vi "DAQmxTasksVI.vi"(8 "error in (no error)":errorcluster, 10 "ControlQueue":refnum<queue>, 11 "DAQmxTaskContainer.lvclass":refnum<class "DAQmxTaskContainer.lvclass">) -> ()   [LabVIEW 2015, in "DAQmxTaskContainer.lvclass"]
uses:
  DAQmxTaskContainer.lvclass
  dependecies/ControlsVIs/Clusters-def/Message types.ctl
  DAQmxTaskContainer.lvclass/DAQmxTaskContainer.ctl
  GeneralFunctionality/GeneralFunctionality.lvclass/GeneralFunctionality.ctl
  Message/Message.lvclass/Message.ctl
  dependecies/ControlsVIs/Clusters-def/Standard Command.ctl
  DAQmxTask.lvclass
  Message/Message.lvclass
  GeneralFunctionality/GeneralFunctionality.lvclass
panel:
  in  "ReInit":bool
  out "Alarm":bool
  in  "divider":i8(knob)=10 min=1 max=20 step=1 scale=1.0..20.0
  out "ELYSE clock pulses":dbl
  out "Received command":string
  in  "DAQmx Tasks":T1(array[cluster])
  out "error out":errorcluster
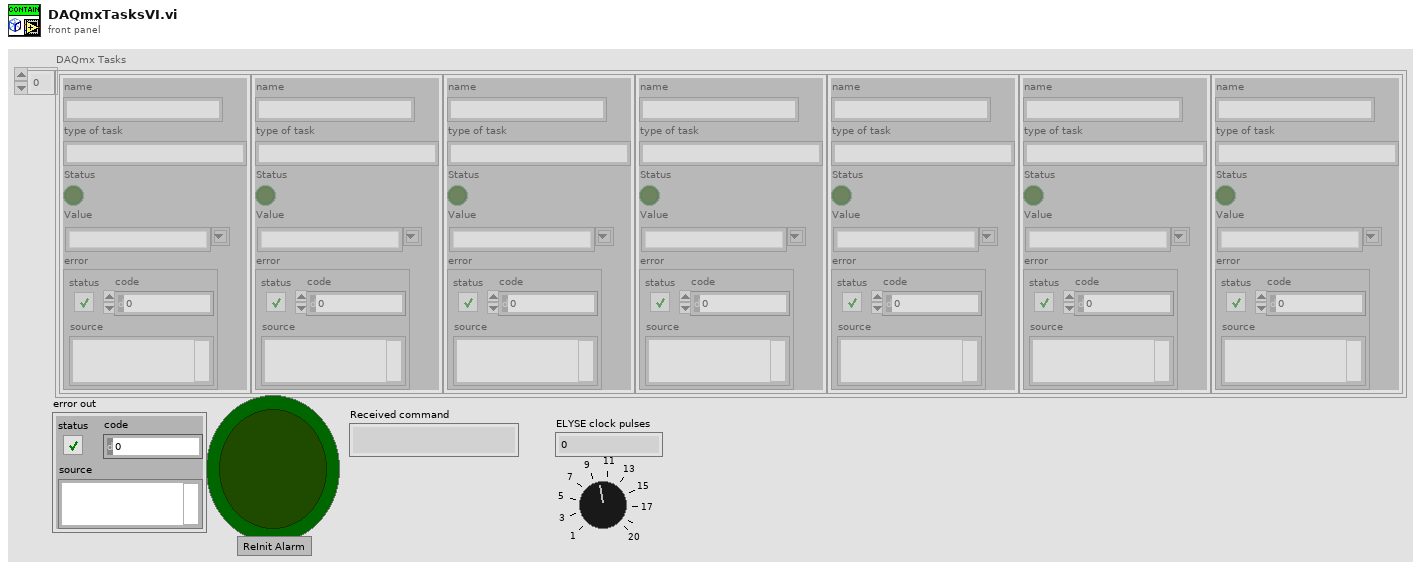
[diagram p1: front panel]
types:
  T1 = cluster{"name":string, "type of task":string, "Status":bool, "Value":string, "error":errorcluster}[]
  T2 = typedef "Message types.ctl" = string
  T3 = typedef "Standard Command.ctl" = cluster{"command":string, "data":variant}
  T4 = cluster{"name":string, "type of task":string, "Status":bool, "Value":string, "error":errorcluster}
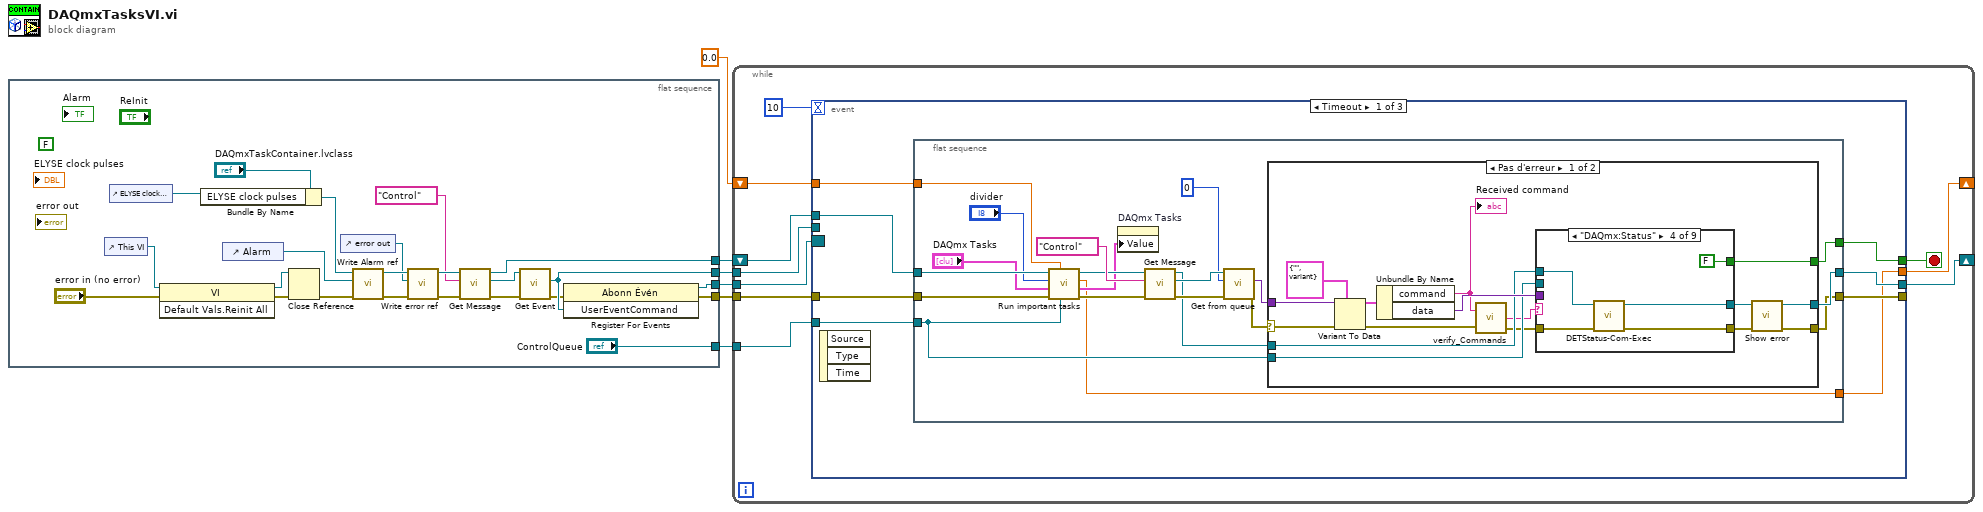
[diagram p0: block diagram]
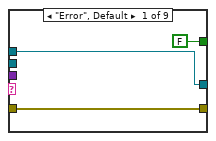
[diagram p2: hidden frame]
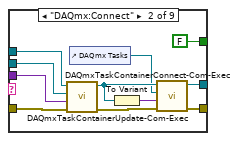
[diagram p3: hidden frame]
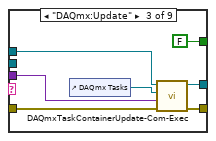
[diagram p4: hidden frame]
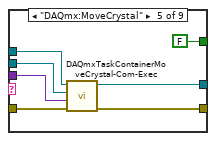
[diagram p5: hidden frame]
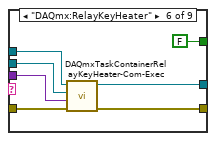
[diagram p6: hidden frame]
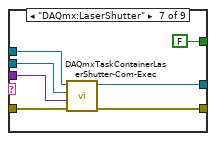
[diagram p7: hidden frame]
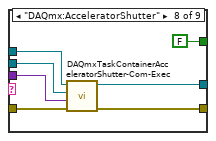
[diagram p8: hidden frame]
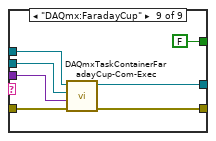
[diagram p9: hidden frame]
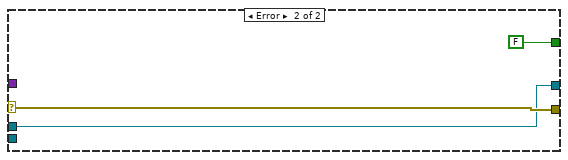
[diagram p10: hidden frame]
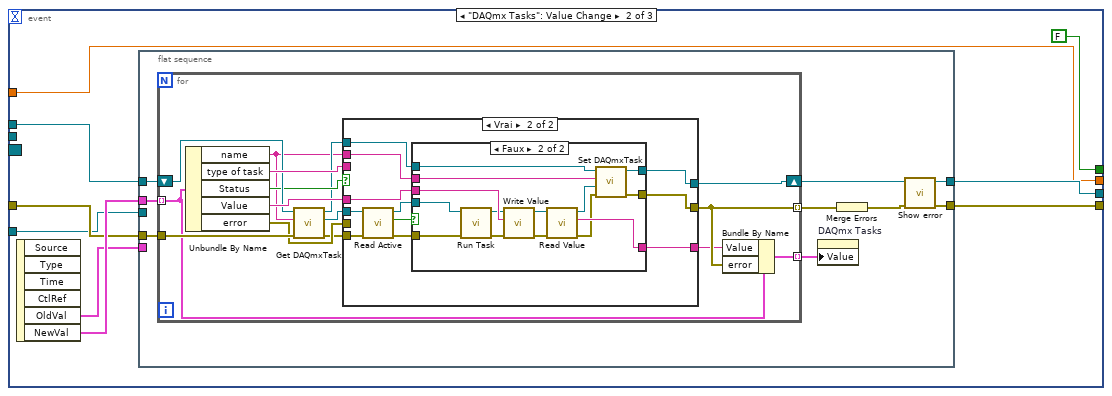
[diagram p11: hidden frame]
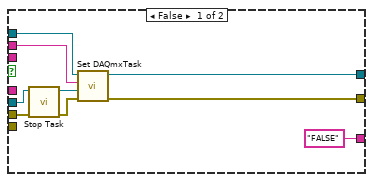
[diagram p12: hidden frame]
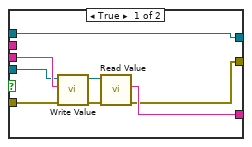
[diagram p13: hidden frame]
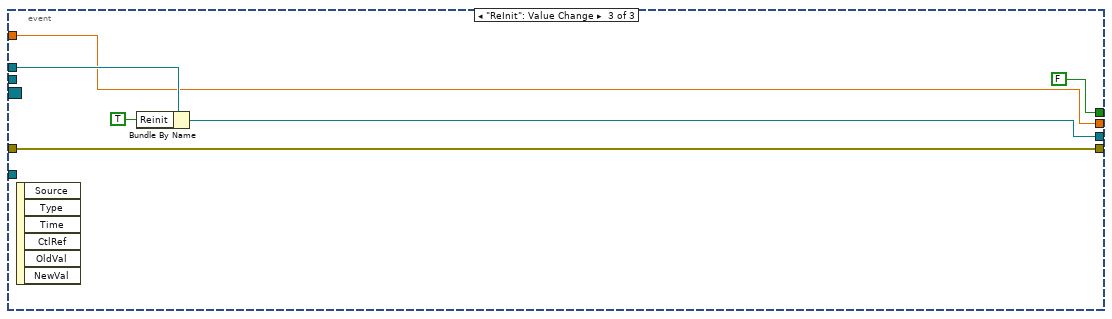
[diagram p14: hidden frame]
diagram:
  n1 = flat-sequence {
    tunnel: [w29] -> w6
    tunnel: [w28] -> w5
    tunnel: ["ControlQueue"] -> w4
    tunnel: [w15] -> w3
    tunnel: [w14] -> w2
    frame #0 {
      (unwired) FALSE ("Clignotant")
      n2 = control-ref of="This VI"() -> (w26:refnum<vi>)
      n3 = control-ref of="ELYSE clock pulses"() -> (w8:refnum<vi>)
      n4 = invoke class="VI" method="Default Vals.Reinit All"(reference=w26, error in="error in (no error)") -> (reference out=w25:refnum<vi>, error out=w27:errorcluster)  [unwired: 1 in, 1 out]
      n5 = Bundle By Name(cluster="DAQmxTaskContainer.lvclass", "ELYSE clock pulses"=w8) -> (w9:refnum<class "DAQmxTaskContainer.lvclass">)
      n6 = control-ref of="Alarm"() -> (w7:refnum<vi>)
      n7 = Close Reference(reference=w25, error in (no error)=w27) -> (error out=w12:errorcluster)
      n8 = control-ref of="error out"() -> (w21:refnum<vi>)
      n9 = call "Write Alarm ref.vi"("error in (no error)"=w12, "Alarm"=w7, "DAQmxTaskContainer in"=w9) -> ("error out"=w23:errorcluster, "DAQmxTaskContainer out"=w22:refnum<class "DAQmxTaskContainer.lvclass">)  [unwired: 7 in]
      n10 = call "Write error ref.vi"("error in (no error)"=w23, "error"=w21, "GeneralFunctionality in"=w22) -> ("error out"=w18:errorcluster, "GeneralFunctionality out"=w17:refnum<class "DAQmxTaskContainer.lvclass">)  [unwired: 7 in]
      n11 = call "Get Message.vi"("error in (no error)"=w18, "Message type"=T2 "Control", "GeneralFunctionality en entrée"=w17) -> ("error out"=w19:errorcluster, "Message.lvclass"=w20:refnum<class "Message.lvclass">, "GeneralFunctionality en sortie"=w14:refnum<class "DAQmxTaskContainer.lvclass">)  [unwired: 6 in]
      n12 = call "Get Event.vi"("error in (no error)"=w19, "Message en entrée"=w20) -> ("error out"=w11:errorcluster, "UserEventCommand"=w15:refnum<user-event>)  [unwired: 7 in, 1 out]
      n13 = register-events(error in=w11, w15) -> (reference out=w29:refnum<event-registration>, error out=w28:errorcluster)  [unwired: 1 in]
    }
  }
  n14 = while {
    tunnel: w6 -> [w39]
    tunnel: w5 -> [w38]
    shift-right: [w36] -> _
    shift-left: w2 -> [w37]
    tunnel: w4 -> [w35]
    tunnel: w3 -> [w33]
    shift-right: [w30] -> _
    shift-left: 0.0 -> [w31]
    stop <- w32 stop-if-true
    n15 = event shown="[0] Timeout" {
      selector: w39 -> [_ _ _]
      dyn-events: _ -> [_ _ _]
      timeout: 10 -> [_ _ _]
      tunnel: [w42 w153 w228] -> _
      tunnel: w38 -> [w44 w155 w228]
      tunnel: w37 -> [w45 w151 w226]
      tunnel: [w43 w152 w225] -> w36
      tunnel: w35 -> [w46 w154 _]
      tunnel: [w47 FALSE ("NewVal") FALSE ("NewVal")] -> w32
      tunnel: w33 -> [_ _ _]
      tunnel: w31 -> [w41 w148 w223]
      tunnel: [w40 w148 w223] -> w30
      event Timeout {
        n16 = event-data() -> ()  [unwired: 1 in, 3 out]
        n17 = flat-sequence {
          tunnel: [w62] -> w47
          tunnel: [w61] -> w43
          tunnel: [w60] -> w42
          tunnel: w46 -> [w53]
          tunnel: w45 -> [w57]
          tunnel: w44 -> [w55]
          tunnel: w41 -> [w49]
          tunnel: [w48] -> w40
          frame #0 {
            n18 = call "Run important tasks.vi"("ControlQueue"=w53, "pulses previous"=w49, "error in (no error)"=w55, "DAQmx Tasks"="DAQmx Tasks", "divider"="divider", "DAQmxTaskContainer in"=w57) -> ("error out"=w54:errorcluster, "DAQmx Tasks out"=w50:T1, "pulses"=w48:dbl, "DAQmxTaskContainer out"=w56:refnum<class "DAQmxTaskContainer.lvclass">)  [unwired: 2 in]
            n19 = property on="DAQmx Tasks" class="Arr (strict)"("Value"=w50) -> ()  [unwired: 2 in, 2 out]
            n20 = call "Get Message.vi"("error in (no error)"=w54, "Message type"=T2 "Control", "GeneralFunctionality en entrée"=w56) -> ("error out"=w67:errorcluster, "Message.lvclass"=w66:refnum<class "Message.lvclass">, "GeneralFunctionality en sortie"=w58:refnum<class "DAQmxTaskContainer.lvclass">)  [unwired: 6 in]
            n21 = call "Get from queue.vi"("error in (no error)"=w67, "timeout in ms (-1)"=0, "Message in"=w66) -> ("error out"=w64:errorcluster, "Data"=w63:variant)  [unwired: 6 in, 1 out]
            n22 = case shown="Pas d'erreur" w64 {
              selector: w64 -> [w81 w146]
              tunnel: w63 -> [w80 _]
              tunnel: [w75 w146] -> w60
              tunnel: [w79 FALSE] -> w62
              tunnel: [w76 w145] -> w61
              tunnel: w58 -> [w77 w145]
              tunnel: w53 -> [w73 _]
              frame No Error {
                n23 = Variant To Data(error in=w81, type=T3 {"command"="", "data"=variant} ("input cluster"), Variant=w80) -> (data=w83:T3, error out=w71:errorcluster)
                n24 = Unbundle By Name(w83) -> ("command"=w68:string, "data"=w78:variant)
                "Received command" <- w68
                n25 = call "verify_Commands.vi"("Command"=w68, "error in"=w71) -> ("Command out"=w69:string, "error out"=w70:errorcluster)  [unwired: 1 out]
                n26 = case shown="\"DAQmx:Status\"" w69 {
                  tunnel: w70 -> [w84 w95 w103 w108 w115 w121 w127 w132 w139]
                  tunnel: [w84 w91 w102 w107 w114 w122 w126 w135 w142] -> w74
                  tunnel: [FALSE FALSE FALSE FALSE FALSE FALSE FALSE FALSE FALSE] -> w79
                  tunnel: [w86 w90 w100 w106 w113 w123 w125 w136 w143] -> w72
                  tunnel: w78 -> [_ w97 w99 _ w116 w120 w128 w133 w140]
                  tunnel: w77 -> [w86 w93 w98 w105 w110 w117 w124 w131 w138]
                  tunnel: w73 -> [_ w96 _ _ w112 w119 w129 w134 w141]
                  frame "Error", Default {
                  }
                  frame "DAQmx:Connect" {
                    n27 = call "DAQmxTaskContainerConnect-Com-Exec.vi"("error in (no error)"=w95, "data"=w97, "ControlQueue"=w96, "DAQmxTaskContainer in"=w93) -> ("error out"=w92:errorcluster, "DAQmxTaskContainer out"=w89:refnum<class "DAQmxTaskContainer.lvclass">)  [unwired: 6 in]
                    n28 = control-ref of="DAQmx Tasks"() -> (w87:refnum<vi>)
                    n29 = To Variant(anything=w89) -> (Variant=w88:variant)
                    n30 = call "DAQmxTaskContainerUpdate-Com-Exec.vi"("error in (no error)"=w92, "data"=w88, "DAQmx Tasks"=w87, "DAQmxTaskContainer in"=w89) -> ("error out"=w91:errorcluster, "DAQmxTaskContainer out"=w90:refnum<class "DAQmxTaskContainer.lvclass">)  [unwired: 6 in]
                  }
                  frame "DAQmx:Update" {
                    n31 = control-ref of="DAQmx Tasks"() -> (w104:refnum<vi>)
                    n32 = call "DAQmxTaskContainerUpdate-Com-Exec.vi"("error in (no error)"=w103, "data"=w99, "DAQmx Tasks"=w104, "DAQmxTaskContainer in"=w98) -> ("error out"=w102:errorcluster, "DAQmxTaskContainer out"=w100:refnum<class "DAQmxTaskContainer.lvclass">)  [unwired: 6 in]
                  }
                  frame "DAQmx:Status" {
                    n33 = call "DETStatus-Com-Exec.vi"("error in (no error)"=w108, "DAQmxTaskContainer in"=w105) -> ("error out"=w107:errorcluster, "DAQmxTaskContainer out"=w106:refnum<class "DAQmxTaskContainer.lvclass">)  [unwired: 8 in]
                  }
                  frame "DAQmx:MoveCrystal" {
                    n34 = call "DAQmxTaskContainerMoveCrystal-Com-Exec.vi"("error in (no error)"=w115, "data"=w116, "ControlQueue"=w112, "DAQmxTaskContainer in"=w110) -> ("error out"=w114:errorcluster, "DAQmxTaskContainer out"=w113:refnum<class "DAQmxTaskContainer.lvclass">)  [unwired: 6 in]
                  }
                  frame "DAQmx:RelayKeyHeater" {
                    n35 = call "DAQmxTaskContainerRelayKeyHeater-Com-Exec.vi"("error in (no error)"=w121, "data"=w120, "ControlQueue"=w119, "DAQmxTaskContainer in"=w117) -> ("error out"=w122:errorcluster, "DAQmxTaskContainer out"=w123:refnum<class "DAQmxTaskContainer.lvclass">)  [unwired: 6 in]
                  }
                  frame "DAQmx:LaserShutter" {
                    n36 = call "DAQmxTaskContainerLaserShutter-Com-Exec.vi"("error in (no error)"=w127, "data"=w128, "ControlQueue"=w129, "DAQmxTaskContainer in"=w124) -> ("error out"=w126:errorcluster, "DAQmxTaskContainer out"=w125:refnum<class "DAQmxTaskContainer.lvclass">)  [unwired: 6 in]
                  }
                  frame "DAQmx:AcceleratorShutter" {
                    n37 = call "DAQmxTaskContainerAcceleratorShutter-Com-Exec.vi"("error in (no error)"=w132, "data"=w133, "ControlQueue"=w134, "DAQmxTaskContainer in"=w131) -> ("error out"=w135:errorcluster, "DAQmxTaskContainer out"=w136:refnum<class "DAQmxTaskContainer.lvclass">)  [unwired: 6 in]
                  }
                  frame "DAQmx:FaradayCup" {
                    n38 = call "DAQmxTaskContainerFaradayCup-Com-Exec.vi"("error in (no error)"=w139, "data"=w140, "ControlQueue"=w141, "DAQmxTaskContainer in"=w138) -> ("error out"=w142:errorcluster, "DAQmxTaskContainer out"=w143:refnum<class "DAQmxTaskContainer.lvclass">)  [unwired: 6 in]
                  }
                }
                n39 = call "Show error.vi"("error in (no error)"=w74, "DAQmxTaskContainer in"=w72) -> ("error out"=w75:errorcluster, "DAQmxTaskContainer out"=w76:refnum<class "DAQmxTaskContainer.lvclass">)  [unwired: 8 in]
              }
              frame Error {
              }
            }
          }
        }
      }
      event "DAQmx Tasks": Value Change {
        n40 = event-data() -> ("OldVal"=w150:T1, "NewVal"=w156:T1)  [unwired: 1 in, 4 out]
        n41 = flat-sequence {
          tunnel: w156 -> [w165]
          tunnel: w155 -> [w164]
          tunnel: w154 -> [_]
          tunnel: [w160] -> w153
          tunnel: [w161] -> w152
          tunnel: w151 -> [w162]
          tunnel: w150 -> [_]
          frame #0 {
            n42 = for {
              tunnel: w165 -> [w171] mode=indexing
              tunnel: w164 -> [w177]
              tunnel: [w169] -> w163 mode=indexing
              shift-right: [w173] -> w157
              shift-left: w162 -> [w178]
              tunnel: [w170] -> w159 mode=indexing
              n43 = Unbundle By Name(w171) -> ("name"=w174:string, "type of task"=w180:string, "Status"=w176:bool, "Value"=w179:string, "error"=w172:errorcluster)
              n44 = call "Get DAQmxTask.vi"("error in (no error)"=w177, "Task name"=w174, "DAQmxTaskContainer in"=w178) -> ("error out"=w166:errorcluster, "DAQmx Task"=w167:refnum<class "DAQmxTask.lvclass">, "DAQmxTaskContainer out"=w175:refnum<class "DAQmxTaskContainer.lvclass">)  [unwired: 6 in]
              n45 = case shown="Vrai" w176 {
                tunnel: w180 -> [_ _]
                tunnel: w179 -> [_ w199]
                tunnel: w172 -> [w189 _]
                tunnel: w175 -> [w187 w191]
                tunnel: w174 -> [w188 w190]
                tunnel: [w186 w192] -> w173
                tunnel: [w185 w198] -> w169
                tunnel: ["FALSE" ("Result") w200] -> w168
                tunnel: w167 -> [w184 w197]
                tunnel: w166 -> [_ w196]
                frame False {
                  n46 = call "Stop Task.vi"("error in (no error)"=w189, "DAQmxTask in"=w184) -> ("error out"=w181:errorcluster, "DAQmxTask out"=w182:refnum<class "DAQmxTask.lvclass">)  [unwired: 8 in]
                  n47 = call "Set DAQmxTask.vi"("error in (no error)"=w181, "DAQmxTask"=w182, "Task name"=w188, "DAQmxTaskContainer in"=w187) -> ("error out"=w185:errorcluster, "DAQmxTaskContainer out"=w186:refnum<class "DAQmxTaskContainer.lvclass">)  [unwired: 6 in]
                }
                frame True {
                  n48 = call-dynamic "Read Active.vi"("error in (no error)"=w196, "DAQmxTask in"=w197) -> ("error out"=w194:errorcluster, "Active?"=w195:bool, "DAQmxTask out"=w193:refnum<class "DAQmxTask.lvclass">)  [unwired: 7 in]
                  n49 = case shown="Faux" w195 {
                    tunnel: [w206 w220] -> w200
                    tunnel: w199 -> [w205 w219]
                    tunnel: [w204 w213] -> w198
                    tunnel: w194 -> [w203 w218]
                    tunnel: w193 -> [w202 w217]
                    tunnel: [w201 w212] -> w192
                    tunnel: w191 -> [w201 w211]
                    tunnel: w190 -> [_ w209]
                    frame True {
                      n50 = call-dynamic "Write Value.vi"("error in (no error)"=w203, "Data"=w205, "DAQmxTask en entrée"=w202) -> ("error out"=w208:errorcluster, "DAQmxTask en sortie"=w207:refnum<class "DAQmxTask.lvclass">)  [unwired: 7 in]
                      n51 = call-dynamic "Read Value.vi"("error in (no error)"=w208, "DAQmxTask en entrée"=w207) -> ("error out"=w204:errorcluster, "Data string"=w206:string)  [unwired: 6 in, 2 out]
                    }
                    frame False {
                      n52 = call "Run Task.vi"("error in (no error)"=w218, "DAQmxTask in"=w217) -> ("error out"=w215:errorcluster, "DAQmxTask out"=w216:refnum<class "DAQmxTask.lvclass">)  [unwired: 8 in]
                      n53 = call-dynamic "Write Value.vi"("error in (no error)"=w215, "Data"=w219, "DAQmxTask en entrée"=w216) -> ("error out"=w222:errorcluster, "DAQmxTask en sortie"=w221:refnum<class "DAQmxTask.lvclass">)  [unwired: 7 in]
                      n54 = call-dynamic "Read Value.vi"("error in (no error)"=w222, "DAQmxTask en entrée"=w221) -> ("error out"=w214:errorcluster, "Data string"=w220:string, "DAQmxTask en sortie"=w210:refnum<class "DAQmxTask.lvclass">)  [unwired: 6 in, 1 out]
                      n55 = call "Set DAQmxTask.vi"("error in (no error)"=w214, "DAQmxTask"=w210, "Task name"=w209, "DAQmxTaskContainer in"=w211) -> ("error out"=w213:errorcluster, "DAQmxTaskContainer out"=w212:refnum<class "DAQmxTaskContainer.lvclass">)  [unwired: 6 in]
                    }
                  }
                }
              }
              n56 = Bundle By Name(cluster=w171, "Value"=w168, "error"=w169) -> (w170:T4)
            }
            n57 = property on="DAQmx Tasks" class="Arr (strict)"("Value"=w159) -> ()  [unwired: 2 in, 2 out]
            n58 = Merge Errors(w163) -> (w158:errorcluster)
            n59 = call "Show error.vi"("error in (no error)"=w158, "DAQmxTaskContainer in"=w157) -> ("error out"=w160:errorcluster, "DAQmxTaskContainer out"=w161:refnum<class "DAQmxTaskContainer.lvclass">)  [unwired: 8 in]
          }
        }
      }
      event "ReInit": Value Change {
        n60 = event-data() -> ()  [unwired: 1 in, 6 out]
        n61 = Bundle By Name(cluster=w226, "Reinit"=TRUE ("AlarmOccured")) -> (w225:refnum<class "DAQmxTaskContainer.lvclass">)
      }
    }
  }
